vi "Validate Simulated Process.vi"(8 "error in (no error)":errorcluster, 11 "URL":refnum<k21>) -> (0 "error out":errorcluster, 2 "Valid?":bool, 3 "dup URL":refnum<k21>)   [LabVIEW 2024]
doc: "Judges whether a URL specifies a valid simulated process."
uses:
  <resource>/objmgr/ni.var.rc
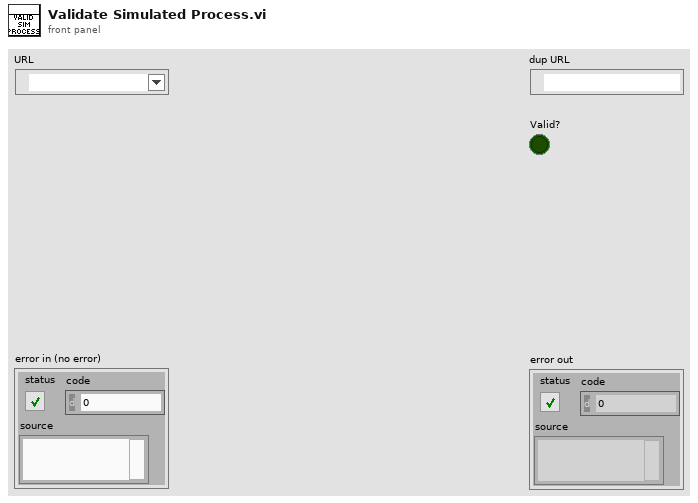
[diagram p1: front panel]
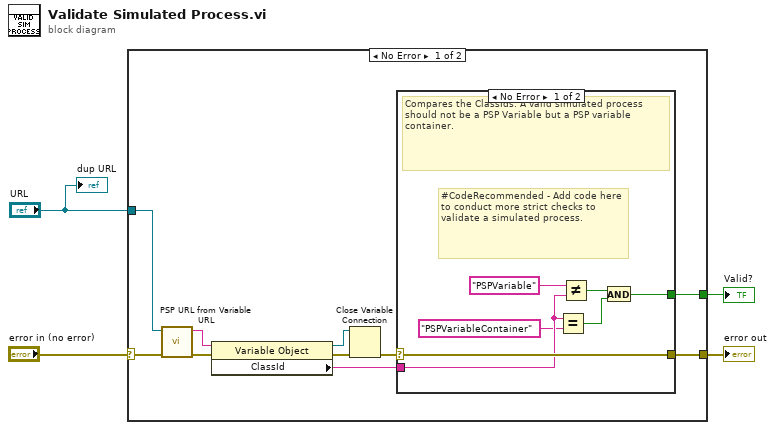
[diagram p0: block diagram]
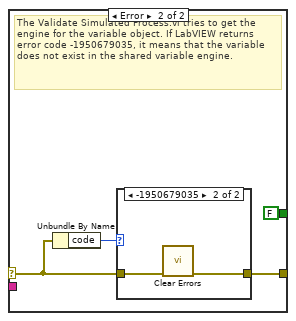
[diagram p2: hidden frame]
diagram:
  n1 = case shown="No Error" "error in (no error)" {
    selector: "error in (no error)" -> [w12 w29]
    tunnel: [w14 w29] -> w4
    tunnel: "URL" -> [w11 _]
    tunnel: [w9 _] -> w2
    frame No Error {
      n2 = call "PSP URL from Variable URL.vi"("error in (no error)"=w12, "Shared Variable URL"=w11) -> ("error out"=w13:errorcluster, "PSP URL"=w10:string)  [unwired: 8 in]
      n3 = property class="Variable Object"(reference=w10, error in=w13) -> (reference out=w8:refnum<k21>, error out=w7:errorcluster, "ClassId"=w5:string)
      n4 = Close Variable Connection(8:w7, 11:w8) -> (0:w6:errorcluster)
      n5 = case shown="No Error" w6 {
        selector: w6 -> [w21 w25]
        tunnel: [w15 FALSE ("Valid?")] -> w9
        tunnel: [w21 w24] -> w14
        tunnel: w5 -> [w19 _]
        frame No Error {
          # "#CodeRecommended - Add code here to conduct more strict checks to validate a simulated process."
          # "Compares the ClassIds. A valid simulated process should not be a PSP Variable but a PSP variable container."
          n6 = Equal?(x=w19, y="PSPVariableContainer" ("x")) -> (x = y?=w16:bool)
          n7 = Not Equal?(x="PSPVariable", y=w19) -> (x != y?=w17:bool)
          n8 = And(x=w17, y=w16) -> (x .and. y?=w15:bool)
        }
        frame Error {
          # "The Validate Simulated Process.vi tries to get the engine for the variable object. If LabVIEW returns error code -1950679035, it means that the variable does not exist in the shared variable engine."
          n9 = Unbundle By Name(w25) -> ("code"=w22:i32)
          n10 = case shown="-1950679035" w22 {
            tunnel: w25 -> [w26 w28]
            tunnel: [w26 w27] -> w24
            frame Default {
            }
            frame -1950679035 {
              n11 = call <vilib>:"Clear Errors.vi"("error in (no error)"=w28) -> ("error out"=w27:errorcluster)  [unwired: 5 in, 1 out]
            }
          }
        }
      }
    }
    frame Error {
    }
  }
  "error out" <- w4
  "Valid?" <- w2
  "dup URL" <- "URL"
